vi "write_attributes.vi"(8 "error in (no error)":errorcluster, 10 "attributes":T1, 11 "BaggingClassifier in":refnum<class "BaggingClassifier.lvclass">) -> (0 "error out":errorcluster, 3 "BaggingClassifier out":refnum<class "BaggingClassifier.lvclass">)   [LabVIEW 2020, in "BaggingClassifier.lvclass"]
uses:
  BaggingClassifier.lvclass
  Controls/bagging_classifier_attributes.ctl
  BaggingClassifier.lvclass/BaggingClassifier.ctl
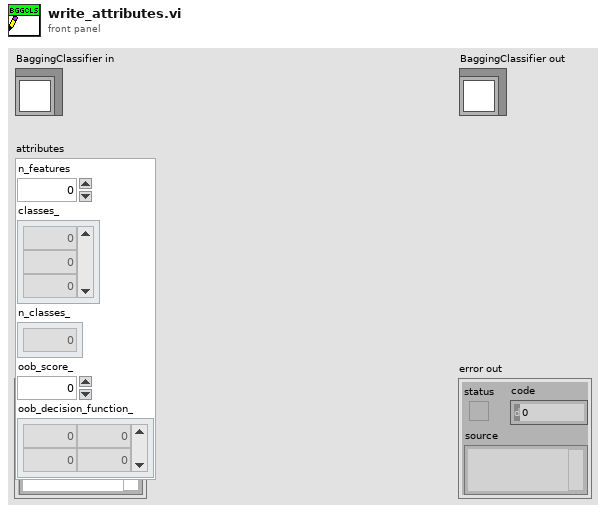
[diagram p1: front panel]
types:
  T1 = typedef "bagging_classifier_attributes.ctl" = cluster{"n_features":dbl, "classes_":dbl[], "n_classes_":dbl[], "oob_score_":dbl, "oob_decision_function_":dbl[][]}
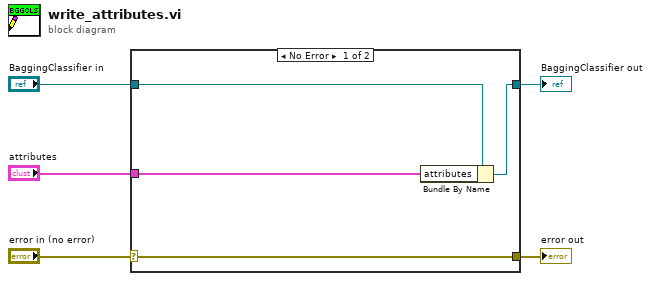
[diagram p0: block diagram]
diagram:
  n1 = case shown="No Error" "error in (no error)" {
    selector: "error in (no error)" -> [w9 w10]
    tunnel: [w9 w10] -> w4
    tunnel: [w7 w11] -> w2
    tunnel: "BaggingClassifier in" -> [w8 w11]
    tunnel: "attributes" -> [w6 _]
    frame No Error {
      n2 = Bundle By Name(cluster=w8, "attributes"=w6) -> (w7:refnum<class "BaggingClassifier.lvclass">)
    }
    frame Error {
    }
  }
  "error out" <- w4
  "BaggingClassifier out" <- w2
